vi "Elevator Launcher.vi"   [LabVIEW 2022 SP3]
uses:
  Elevator Controller Actor/Elevator Controller Actor/Elevator Controller Actor.lvclass
  C:/Program Files/National Instruments/LabVIEW 2022/vi.lib/ActorFramework/Actor/Actor.lvclass
  Elevator Controller Actor/Elevator Controller Actor/State -Enum.ctl
  Interface Elevator/Interface Elevator Msg/Set State Msg/Set State Msg.lvclass/Set State Msg.ctl
  <vilib>/ActorFramework/Message Enqueuer/Message Enqueuer.lvclass/Message Enqueuer.ctl
  <vilib>/ActorFramework/Message Enqueuer/Enqueue.vi
  Interface Elevator/Interface Elevator Msg/Set State Msg/Set State Msg.lvclass
  C:/Program Files/National Instruments/LabVIEW 2022/vi.lib/ActorFramework/Message/Message.lvclass
  <vilib>/ActorFramework/Message Priority Queue/Priority Enqueue.vi
  <vilib>/ActorFramework/Actor/Actor.lvclass
panel:
  # "[Covers: SI1]"
types:
  T1 = typedef "Elevator Controller Actor.lvlib/Elevator Controller Actor.lvclass/State -Enum.ctl" = enum16{"Initial", "Wait for First Request", "Start and Move", "Anaysis", "Continue Travel", "Stop at Floor", "Open and Close Door Sequence", "No Request Remaining", "Emergency Call", "Terminate Process"}
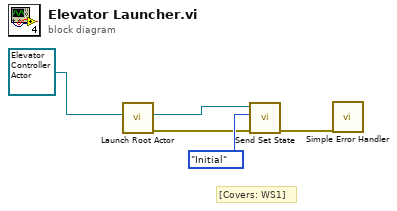
[diagram p0: block diagram]
diagram:
  # "[Covers: WS1]"
  n1 = call <vilib>:"Launch Root Actor.vi"("Actor"=refnum<class "Elevator Controller Actor.lvclass"> refnum ("Elevator Controller Actor.lvlib:Elevator Controller Actor.lvclass")) -> ("error out"=w2:errorcluster, "Actor's Enqueuer"=w4:refnum<class "Message Enqueuer.lvclass">)  [unwired: 9 in]
  n2 = call "Send Set State.vi"("error in (no error)"=w2, "State"=State_-Enum."Initial", "Message Enqueuer"=w4) -> ("error out"=w1:errorcluster)  [unwired: 7 in, 1 out]
  n3 = call <vilib>:"Simple Error Handler.vi"("error in (no error)"=w1) -> ()  [unwired: 4 in, 5 out]
